vi "PDC_MRAWFileLoad.vi"(6 "MRawBitDepth":u32, 8 "error in (no error)":errorcluster, 9 "ImageBuffInfo":T1, 10 "FrameNo":i32, 11 "FileNo":u32) -> (0 "error out":errorcluster, 2 "ErrorCode":u32, 3 "ReturnValue":u32, 4 "Data(8Bit)":u8[](array[numeric]), 5 "Data(16Bit)":u16[](array[numeric]))   [LabVIEW 8.6]
doc: "This VI acquires image data of specified frame from opened MRAW file."
uses:
  PDCLIB.dll
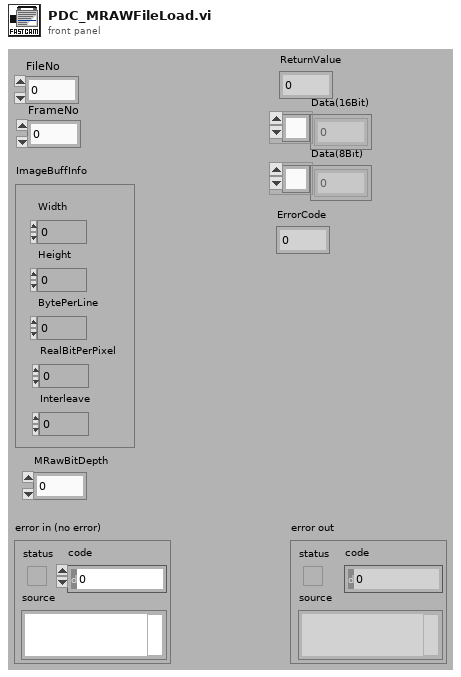
[diagram p1: front panel]
types:
  T1 = cluster{"Width":i32, "Height":i32, "BytePerLine":i32, "RealBitPerPixel":u16, "Interleave":i32}
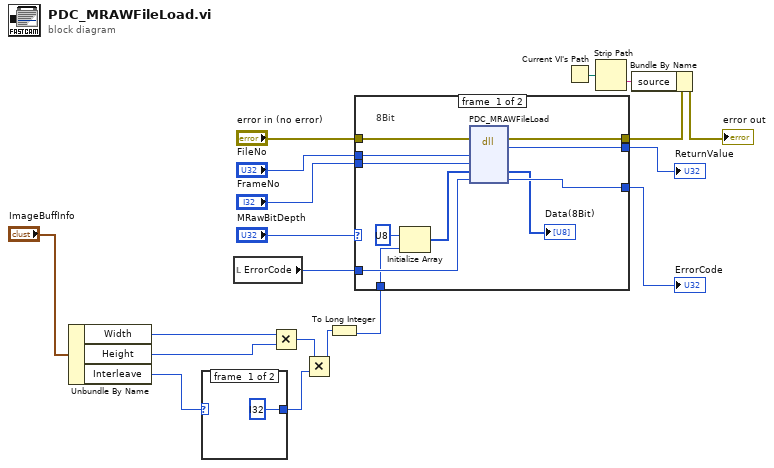
[diagram p0: block diagram]
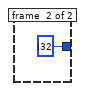
[diagram p2: hidden frame]
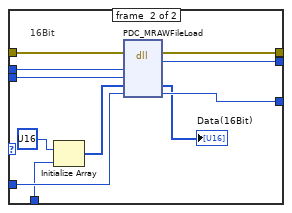
[diagram p3: hidden frame]
diagram:
  n1 = Unbundle By Name("ImageBuffInfo") -> ("Width"=w10:i32, "Height"=w9:i32, "Interleave"=w2:i32)
  n2 = case shown="1, 2" w2 {
    tunnel: [i32 ? ("y") i32 ? ("y")] -> w12
    frame #0 {
    }
    frame #1 {
    }
  }
  n3 = local read "ErrorCode"() -> (w17:u32)
  n4 = Multiply(x=w10, y=w9) -> (x*y=w13:i32)
  n5 = Multiply(x=w13, y=w12) -> (x*y=w11:i32)
  n6 = To Long Integer(number=w11) -> (32bit integer=w4:i32)
  n7 = case shown="1..3" "MRawBitDepth" {
    tunnel: [w32 w43] -> w19
    tunnel: [w31 w42] -> w6
    tunnel: "error in (no error)" -> [w30 w41]
    tunnel: w17 -> [w29 w40]
    tunnel: "FileNo" -> [w28 w39]
    tunnel: "FrameNo" -> [w27 w38]
    tunnel: [w26 w37] -> w14
    tunnel: w4 -> [w23 w34]
    frame #0 {
      # "8Bit"
      n8 = Initialize Array(u8 ? ("要素"), w23) -> (w22:u8[])
      n9 = dll-call lib="PDCLIB.dll" fn="PDC_MRAWFileLoad"(error in=w30, "nFileNo"=w28, "nFrameNo"=w27, "pBuff"=w22, "pErrorCode"=w29) -> (error out=w31:errorcluster, "return type"=w32:u32, "pBuff"=→"Data(8Bit)":u8[], "pErrorCode"=w26:u32)  [unwired: 4 in, 1 out]
    }
    frame #1 {
      # "16Bit"
      n10 = Initialize Array(u16 ? ("要素"), w34) -> (w33:u16[])
      n11 = dll-call lib="PDCLIB.dll" fn="PDC_MRAWFileLoad"(error in=w41, "nFileNo"=w39, "nFrameNo"=w38, "pData"=w33, "pErrorCode"=w40) -> (error out=w42:errorcluster, "return type"=w43:u32, "pData"=→"Data(16Bit)":u16[], "pErrorCode"=w37:u32)  [unwired: 4 in, 1 out]
    }
  }
  "ReturnValue" <- w19
  "ErrorCode" <- w14
  n12 = Current VI's Path() -> (path=w7:path)
  n13 = Strip Path(path=w7) -> (name=w8:string)  [unwired: 1 out]
  n14 = Bundle By Name(cluster=w6, "source"=w8) -> (→"error out":errorcluster)
